vi "LaunchHelp.vi"(10 "Help Topic":string, 11 "Help File":string) -> ()   [LabVIEW 2021]
uses:
  <vilib>/Platform/browser.llb/Open URL in Default Browser (string).vi
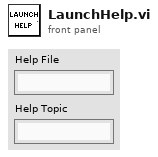
[diagram p1: front panel]
types:
  T1 = enum32{"invalid OS target", "Mac OS", "Windows 3.1", "Windows 95/NT", "Solaris 1", "Solaris 2", "HP-UX", "PowerMAX", "Linux", "Irix", "Rhapsody", "BeOS", "AIX", "OSF1", "VxWorks", "PharLap", "Carbon", "RTX", "Windows x64", "Linux x64", "Mac OS X x64"}
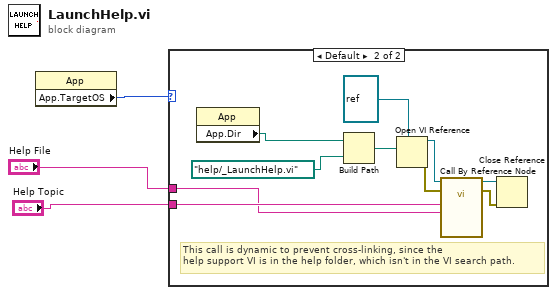
[diagram p0: block diagram]
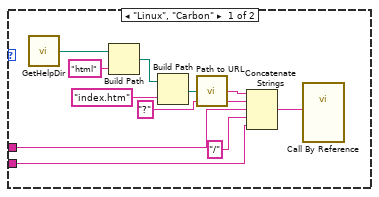
[diagram p2: hidden frame]
diagram:
  n1 = property on="Property Node" class="App"() -> ("App.TargetOS"=w3:T1)  [unwired: 2 in, 2 out]
  n2 = case shown="Default" w3 {
    tunnel: "Help File" -> [w5 w18]
    tunnel: "Help Topic" -> [w10 w19]
    frame "Linux", "Carbon" {
      n3 = call <vilib>:"GetHelpDir.vi"() -> ("help path"=w9:path)
      n4 = Build Path(base path=w9, name or relative path="html") -> (appended path=w13:path)
      n5 = Build Path(base path=w13, name or relative path="index.htm") -> (appended path=w12:path)
      n6 = call <vilib>:"Path to URL.vi"("path"=w12) -> ("url"=w11:string)
      n7 = Concatenate Strings(w11, "?" ("string"), w5, "/" ("string"), w10) -> (w4:string)
      n8 = call-by-ref "?"("URL"=w4) -> ()  [unwired: 7 in, 4 out]
    }
    frame Default {
      # "This call is dynamic to prevent cross-linking, since the\nhelp support VI is in the help folder, which isn't in the VI search path."
      n9 = property on="Property Node" class="App"() -> ("App.Dir"=w23:path)  [unwired: 2 in, 2 out]
      n10 = Build Path(base path=w23, name or relative path=path "help/_LaunchHelp.vi") -> (appended path=w22:path)
      n11 = Open VI Reference(type specifier VI Refnum (for type only)=refnum<vi> refnum, vi path=w22) -> (vi reference=w21:refnum<vi>, error out=w17:errorcluster)  [unwired: 4 in]
      n12 = call-by-ref "Call By Reference Node"(reference=w21, error in=w17, "CHM or HLP filename (lvdialog.chm)"=w18, "HTML filename"=w19) -> (reference out=w15:refnum<vi>, error out=w16:errorcluster)  [unwired: 5 in, 1 out]
      n13 = Close Reference(reference=w15, error in (no error)=w16) -> ()  [unwired: 1 out]
    }
  }
